vi "Serial Read.vi"(8 "error in":errorcluster, 9 "timeout (ms)":i32, 10 "bytes to read":i32, 11 "Visa Resource":refnum<visa-resource-name>) -> (0 "error out":errorcluster, 1 "timed out?":bool, 3 "data":u8[](array[numeric]))   [LabVIEW 2021, in "Serial Shared Components.lvlib"]
doc: "Performs a read on the serial port."
uses:
  Serial Shared Components.lvlib
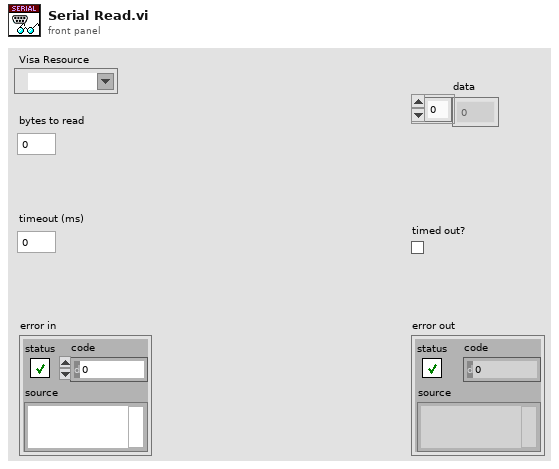
[diagram p1: front panel]
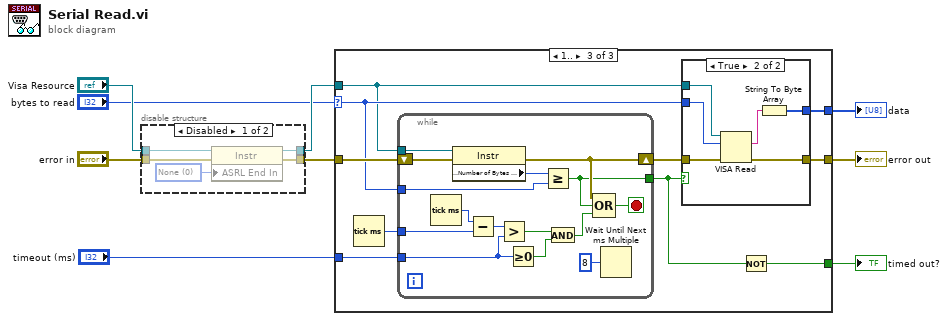
[diagram p0: block diagram]
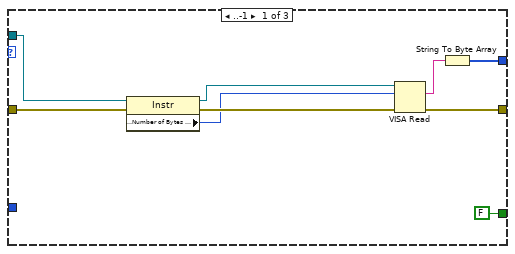
[diagram p3: hidden frame]
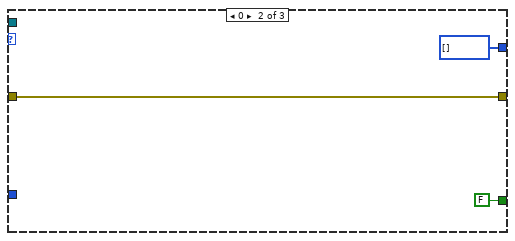
[diagram p4: hidden frame]
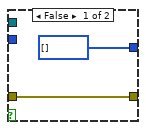
[diagram p5: hidden frame]
diagram:
  n1 = disable-structure shown="Disabled" {
    disable-tunnel: "error in" -> [w14 w15]
    disable-tunnel: "Visa Resource" -> [w13 w16]
    disable-tunnel: [w11 w16] -> w4
    disable-tunnel: [w10 w15] -> w2
    frame Disabled {
      w12 = u16 0 items=["None", "Last Bit", "TermChar"] ("Serial Settings:End Mode for Reads")
      n2 = property class="Instr"(reference=w13, error in=w14, "ASRL End In"=w12) -> (reference out=w11:refnum<visa-resource-name>, error out=w10:errorcluster)
    }
    frame Enabled {
    }
  }
  n3 = case shown="1.." "bytes to read" {
    selector: "bytes to read" -> [_ _ w35]
    tunnel: "timeout (ms)" -> [_ _ w33]
    tunnel: w2 -> [w25 w27 w38]
    tunnel: w4 -> [w24 _ w34]
    tunnel: [w20 w27 w37] -> w6
    tunnel: [w17 u8[] [] ("unsigned byte array") w36] -> w7
    tunnel: [FALSE FALSE w32] -> w5
    frame ..-1 {
      n4 = property class="Instr"(reference=w24, error in=w25) -> (reference out=w22:refnum<visa-resource-name>, error out=w23:errorcluster, "Serial Settings:Number of Bytes at Serial Port"=w21:u32)
      n5 = VISA Read(VISA resource name=w22, byte count=w21, error in (no error)=w23) -> (read buffer=w18:string, error out=w20:errorcluster)  [unwired: 2 out]
      n6 = String To Byte Array(string=w18) -> (unsigned byte array=w17:u8[])
    }
    frame 0 {
    }
    frame 1.. {
      n7 = Tick Count (ms)() -> (millisecond timer value=w31:u32)
      n8 = while {
        tunnel: w31 -> [w53]
        shift-right: [w57] -> w30
        shift-left: w38 -> [w61]
        tunnel: w35 -> [w58]
        tunnel: w34 -> [w60]
        tunnel: [w56] -> w29
        tunnel: w33 -> [w49]
        stop <- w55 stop-if-true
        n9 = Tick Count (ms)() -> (millisecond timer value=w54:u32)
        n10 = property class="Instr"(reference=w60, error in=w61) -> (error out=w57:errorcluster, "Serial Settings:Number of Bytes at Serial Port"=w59:u32)  [unwired: 1 out]
        n11 = Subtract(x=w54, y=w53) -> (x-y=w51:u32)
        n12 = Greater?(x=w51, y=w49) -> (0:w50:bool)
        n13 = Greater Or Equal To 0?(x=w49) -> (x >= 0?=w48:bool)
        n14 = Greater Or Equal?(x=w59, y=w58) -> (x >= y?=w56:bool)
        n15 = And(x=w50, y=w48) -> (x .and. y?=w52:bool)
        n16 = Compound Arithmetic op=OR(w57, w56, w52) -> (w55:bool)
        n17 = Wait Until Next ms Multiple(millisecond multiple=u32 8) -> ()  [unwired: 1 out]
      }
      n18 = case shown="True" w29 {
        tunnel: w34 -> [_ w44]
        tunnel: w30 -> [w39 w46]
        tunnel: [w39 w45] -> w37
        tunnel: [u8[] [] ("data") w42] -> w36
        tunnel: w35 -> [_ w43]
        frame False {
        }
        frame True {
          n19 = VISA Read(VISA resource name=w44, byte count=w43, error in (no error)=w46) -> (read buffer=w41:string, error out=w45:errorcluster)  [unwired: 2 out]
          n20 = String To Byte Array(string=w41) -> (unsigned byte array=w42:u8[])
        }
      }
      n21 = Not(x=w29) -> (.not. x?=w32:bool)
    }
  }
  "error out" <- w6
  "data" <- w7
  "timed out?" <- w5
